vi "Add CANBus Received Frames.vi"(8 "error in (no error)":errorcluster, 10 "CAN Frames":T1[](array[typedef]) {"payload" format="%x"; "timestamp" format="%<%.7X\n%x>T"; "type" items=["CAN Data"=0, "CAN Remote"=1, "CAN Bus Error"=2, "CAN 2.0 Data"=8, "CAN FD Data"=16, "CAN FD+BRS Data"=24, "J1939 Data"=192, "Delay"=224, "Log Trigger"=225, "Start Trigger"=226]; "identifier" format="%x"}, 11 "Load Calculator in":refnum<class "GenBus_Load_Calculator.lvclass">) -> (0 "error out":errorcluster, 3 "Load Calculator out":refnum<class "GenBus_Load_Calculator.lvclass">)   [LabVIEW 2019, in "XNET-Bus-Load-Calculator.lvlib"]
uses:
  XNET-Bus-Load-Calculator.lvlib
  GenBus/GenBus_Load_Calculator.lvclass
  <vilib>/xnet/xnet.llb/XNET Frame CAN.ctl
  <vilib>/xnet/xnet.llb/XNET Frame Type CAN.ctl
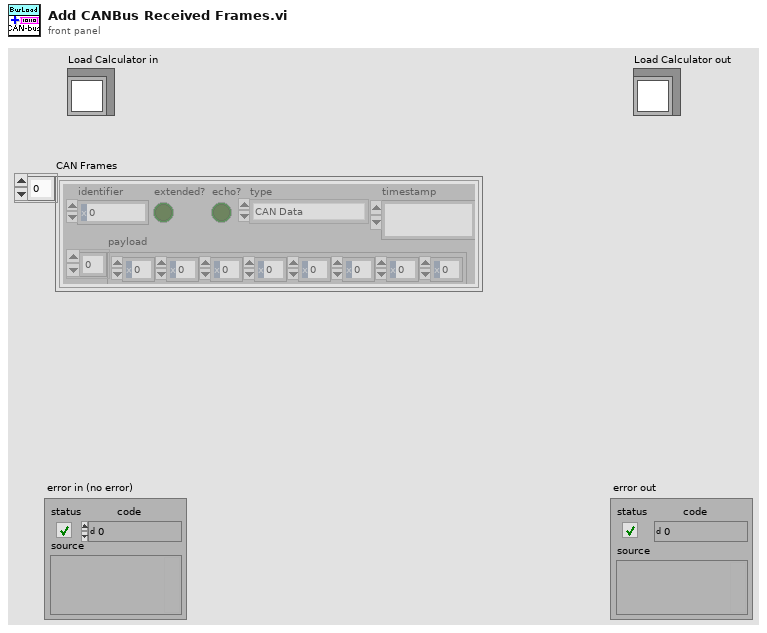
[diagram p1: front panel]
types:
  T1 = typedef "XNET Frame CAN.ctl" = cluster{"timestamp":timestamp, "payload":u8[], "identifier":u32, "type":T2, "extended?":bool, "echo?":bool}
  T2 = typedef "XNET Frame Type CAN.ctl" = u8
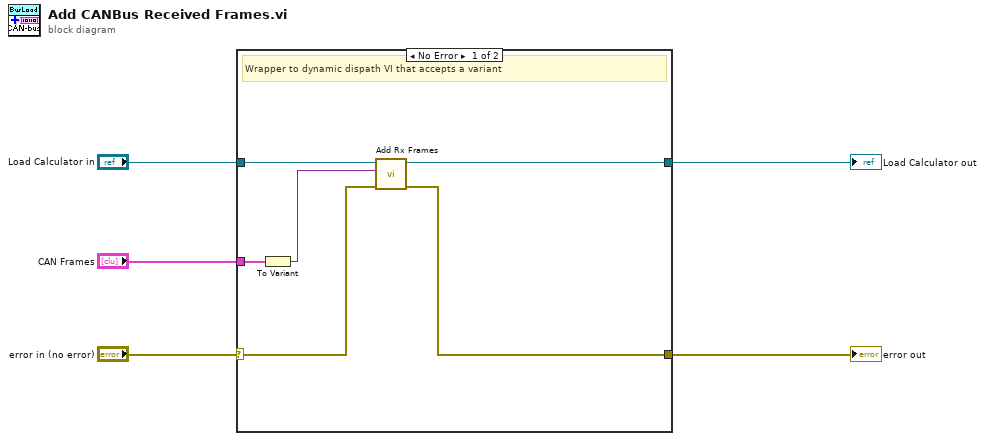
[diagram p0: block diagram]
diagram:
  n1 = case shown="No Error" "error in (no error)" {
    selector: "error in (no error)" -> [w9 w13]
    tunnel: [w6 w13] -> w4
    tunnel: "CAN Frames" -> [w8 _]
    tunnel: "Load Calculator in" -> [w11 w12]
    tunnel: [w10 w12] -> w1
    frame No Error {
      # "Wrapper to dynamic dispath VI that accepts a variant"
      n2 = To Variant(anything=w8) -> (Variant=w7:variant)
      n3 = call-dynamic "Add Rx Frames.vi"("error in (no error)"=w9, "Frames"=w7, "GenBus_Load_Calculator in"=w11) -> ("error out"=w6:errorcluster, "GenBus_Load_Calculator out"=w10:refnum<class "GenBus_Load_Calculator.lvclass">)  [unwired: 7 in]
    }
    frame Error {
    }
  }
  "error out" <- w4
  "Load Calculator out" <- w1
